vi "ProdaNG.Tree.GetAll.vi"(7 "TestStepsTree":refnum<vi>, 8 "error in (no error)":errorcluster) -> (0 "error out":errorcluster, 1 "Selected elements values":T1[](array[typedef]), 2 "Selected elements":T2[](array[typedef]))   [LabVIEW 2016]
uses:
  ProdaNG.Tree.Fglb.Data.ctl
  ProdaNG.Tree.Fglb.Element.ctl
  ProdaNG.Tree.Fglb.Value.ctl
  ProdaNG.Tree.Fglb.Action.ctl
  ProdaNG.Configurator.Glb.vi
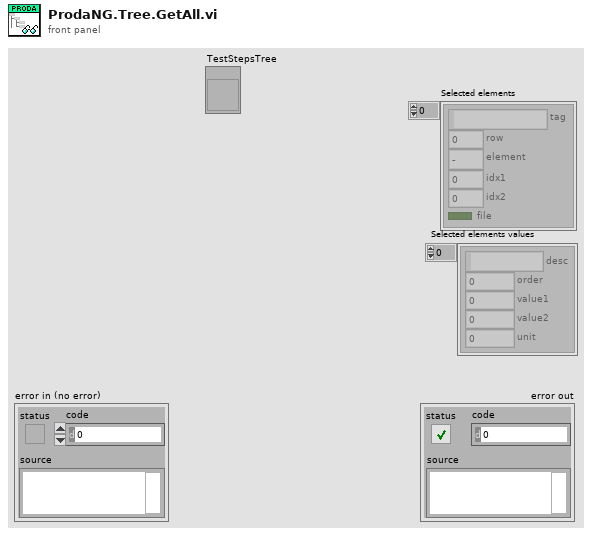
[diagram p1: front panel]
types:
  T1 = typedef "ProdaNG.Tree.Fglb.Value.ctl" = cluster{"desc":string, "order":i32, "value1":dbl, "value2":dbl, "unit":i32}
  T2 = typedef "ProdaNG.Tree.Fglb.Data.ctl" = cluster{"tag":string, "row":i32, "element":T3, "idx1":i32, "idx2":i32, "file":bool}
  T3 = typedef "ProdaNG.Tree.Fglb.Element.ctl" = enum16{"-", "PP", "TS", "TP", "TV"}
  T4 = typedef "ProdaNG.Tree.Fglb.Action.ctl" = enum16{"init", "add", "get by row", "get by tag", "get by idx"}
  T5 = typedef "ProdaNG.ProcessStepParam.ctl" = cluster{"i_id":i32, "processStepId":i32, "unitId":i32, "contentId":string, "previewId":string, "value":dbl, "valueText":string, "paramSequence":i32, "history":i32, "mdReason":string, "mdUser":string, "mdTime":string, "description":string}
  T6 = cluster{"description":string, "paramSequence":i32, "value":dbl, dbl, "unitId":i32}
  T7 = typedef "ProdaNG.TestStep.ctl" = cluster{"i_id":i32, "processStepId":i32, "testSequence":i32, "testOrder":i32, "mdReason":string, "mdUser":string, "mdTime":string, "description":string}
  T8 = typedef "ProdaNG.TestStepParam.ctl" = cluster{"i_id":i32, "testStepId":i32, "unitId":i32, "contentId":string, "previewId":string, "value":dbl, "valueText":string, "paramSequence":i32, "history":i32, "mdReason":string, "mdUser":string, "mdTime":string, "description":string}
  T9 = typedef "ProdaNG.TestValue.ctl" = cluster{"i_id":i32, "testStepId":i32, "releaseId":i32, "unitId":i32, "contentId":string, "previewId":string, "maximum":dbl, "minimum":dbl, "valueText":string, "testValueSequence":i32, "history":i32, "mdReason":string, "mdUser":string, "mdTime":string, "description":string}
  T10 = cluster{"description":string, "testSequence":i32, dbl, dbl, "unitId":i32}
  T11 = cluster{"description":string, "testValueSequence":i32, "minimum":dbl, "maximum":dbl, "unitId":i32}
  T12 = cluster{"element":T3, "found entry":T2, cluster{"description":string, "testValueSequence":i32, "minimum":dbl, "maximum":dbl, "unitId":i32}}
  T13 = cluster{"element":T3, "found entry":T2, cluster{"description":string, "testValueSequence":i32, "minimum":dbl, "maximum":dbl, "unitId":i32}}[]
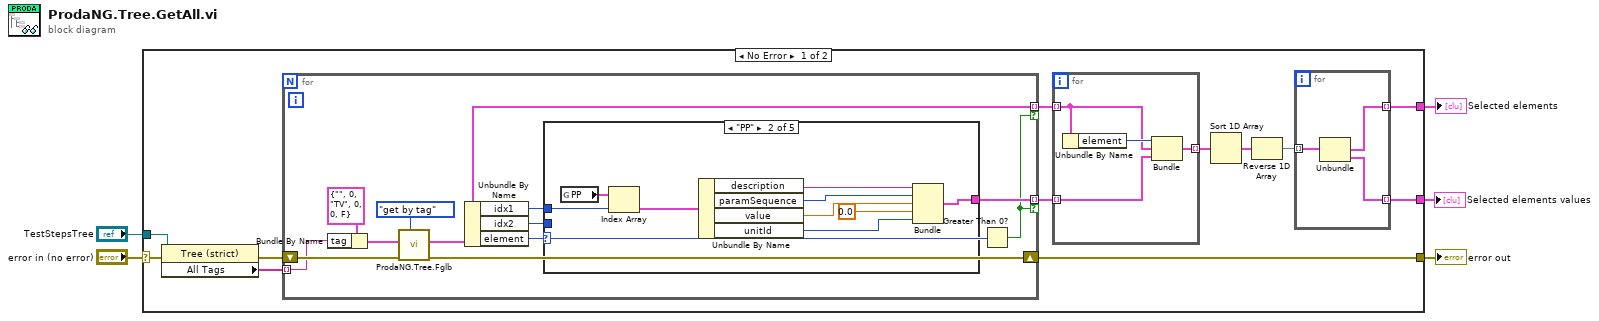
[diagram p0: block diagram]
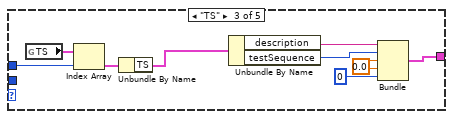
[diagram p3: hidden frame]
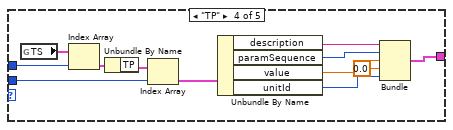
[diagram p4: hidden frame]
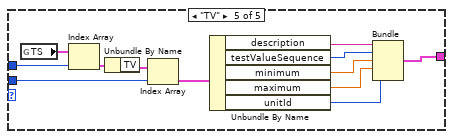
[diagram p5: hidden frame]
diagram:
  n1 = case shown="No Error" "error in (no error)" {
    selector: "error in (no error)" -> [w17 w79]
    tunnel: "TestStepsTree" -> [w14 _]
    tunnel: [w15 w79] -> w5
    tunnel: [w9 _] -> w2
    tunnel: [w7 _] -> w1
    frame No Error {
      n2 = property on="Property Node" class="Tree (strict)"(reference=w14, error in=w17) -> (error out=w16:errorcluster, "All Tags"=w6:string[])  [unwired: 1 out]
      n3 = for {
        shift-right: [w31] -> w15
        shift-left: w16 -> [w33]
        tunnel: [w32] -> w10 mode=indexing if=w26
        tunnel: [w28] -> w8 mode=indexing if=w26
        tunnel: w6 -> [w25] mode=indexing
        n4 = Bundle By Name(cluster=T2 {"tag"="", "row"=0, "element"=enum."TV", "idx1"=0, "idx2"=0, "file"=FALSE} ("entry in"), "tag"=w25) -> (w34:T2)
        n5 = call "ProdaNG.Tree.Fglb.vi"("Action (add)"=ProdaNG.Tree.Fglb.Action."get by tag", "error in"=w33, "entry in"=w34) -> ("error out"=w31:errorcluster, "found entry"=w32:T2)  [unwired: 6 in, 1 out]
        n6 = Unbundle By Name(w32) -> ("idx1"=w29:i32, "idx2"=w30:i32, "element"=w27:T3)
        n7 = case shown="\"PP\"" w27 {
          tunnel: w30 -> [_ _ _ w63 w75]
          tunnel: w29 -> [_ w42 w51 w62 w74]
          tunnel: [_ w40 w48 w58 w70] -> w28
          frame "-" {
          }
          frame "PP" {
            n8 = global read "ProdaNG.Configurator.Glb.vi" "PP"() -> (w45:T5[])
            n9 = Index Array(array=w45, index=w42) -> (element=w41:T5)
            n10 = Unbundle By Name(w41) -> ("description"=w44:string, "paramSequence"=w43:i32, "value"=w39:dbl, "unitId"=w37:i32)
            n11 = Bundle("description"=w44, "paramSequence"=w43, "value"=w39, 0.0, "unitId"=w37) -> (w40:T6)  [unwired: 1 in]
          }
          frame "TS" {
            w49 = 0.0
            n12 = global read "ProdaNG.Configurator.Glb.vi" "TS"() -> (w54:cluster{"TS":T7, "TP":T8[], "TV":T9[]}[])
            n13 = Index Array(array=w54, index=w51) -> (element=w50:cluster{"TS":T7, "TP":T8[], "TV":T9[]})
            n14 = Unbundle By Name(w50) -> ("TS"=w47:T7)
            n15 = Unbundle By Name(w47) -> ("description"=w53:string, "testSequence"=w52:i32)
            n16 = Bundle("description"=w53, "testSequence"=w52, w49, w49, "unitId"=0) -> (w48:T10)  [unwired: 1 in]
          }
          frame "TP" {
            n17 = global read "ProdaNG.Configurator.Glb.vi" "TS"() -> (w66:cluster{"TS":T7, "TP":T8[], "TV":T9[]}[])
            n18 = Index Array(array=w66, index=w62) -> (element=w65:cluster{"TS":T7, "TP":T8[], "TV":T9[]})
            n19 = Unbundle By Name(w65) -> ("TP"=w64:T8[])
            n20 = Index Array(array=w64, index=w63) -> (element=w61:T8)
            n21 = Unbundle By Name(w61) -> ("description"=w60:string, "paramSequence"=w59:i32, "value"=w57:dbl, "unitId"=w55:i32)
            n22 = Bundle("description"=w60, "paramSequence"=w59, "value"=w57, 0.0, "unitId"=w55) -> (w58:T6)  [unwired: 1 in]
          }
          frame "TV" {
            n23 = global read "ProdaNG.Configurator.Glb.vi" "TS"() -> (w78:cluster{"TS":T7, "TP":T8[], "TV":T9[]}[])
            n24 = Index Array(array=w78, index=w74) -> (element=w77:cluster{"TS":T7, "TP":T8[], "TV":T9[]})
            n25 = Unbundle By Name(w77) -> ("TV"=w76:T9[])
            n26 = Index Array(array=w76, index=w75) -> (element=w73:T9)
            n27 = Unbundle By Name(w73) -> ("description"=w72:string, "testValueSequence"=w71:i32, "minimum"=w69:dbl, "maximum"=w68:dbl, "unitId"=w67:i32)
            n28 = Bundle("description"=w72, "testValueSequence"=w71, "minimum"=w69, "maximum"=w68, "unitId"=w67) -> (w70:T11)  [unwired: 1 in]
          }
        }
        n29 = Greater Than 0?(x=w27) -> (x > 0?=w26:bool)
      }
      n30 = for {
        tunnel: w10 -> [w23] mode=indexing
        tunnel: w8 -> [w21] mode=indexing
        tunnel: [w22] -> w13 mode=indexing
        n31 = Unbundle By Name(w23) -> ("element"=w24:T3)
        n32 = Bundle("element"=w24, "found entry"=w23, w21) -> (w22:T12)  [unwired: 1 in]
      }
      n33 = Sort 1D Array(array=w13) -> (sorted array=w12:T13)
      n34 = Reverse 1D Array(array=w12) -> (reversed array=w11:T13)
      n35 = for {
        tunnel: w11 -> [w20] mode=indexing
        tunnel: [w19] -> w9 mode=indexing
        tunnel: [w18] -> w7 mode=indexing
        n36 = Unbundle(w20) -> ("found entry"=w19:T2, w18:T11)  [unwired: 1 out]
      }
    }
    frame Error {
    }
  }
  "error out" <- w5
  "Selected elements" <- w2
  "Selected elements values" <- w1
